vi "rad_Format Image Results.vi"(7 "Results listbox":refnum<vi>, 8 "error in (no error)":errorcluster, 10 "AppImage 2":T1, 11 "AppImage 1":T1) -> (0 "error out":errorcluster)   [LabVIEW 2016]
uses:
  App Images/TypeDefs/rad_Application Image Properties.ctl
  App Images/TypeDefs/rad_FPGA Properties.ctl
  App Images/TypeDefs/rad_FPGA Flash Properties.ctl
  <vilib>/Utility/miscctls.llb/LVRowAndColumnTypeDef.ctl
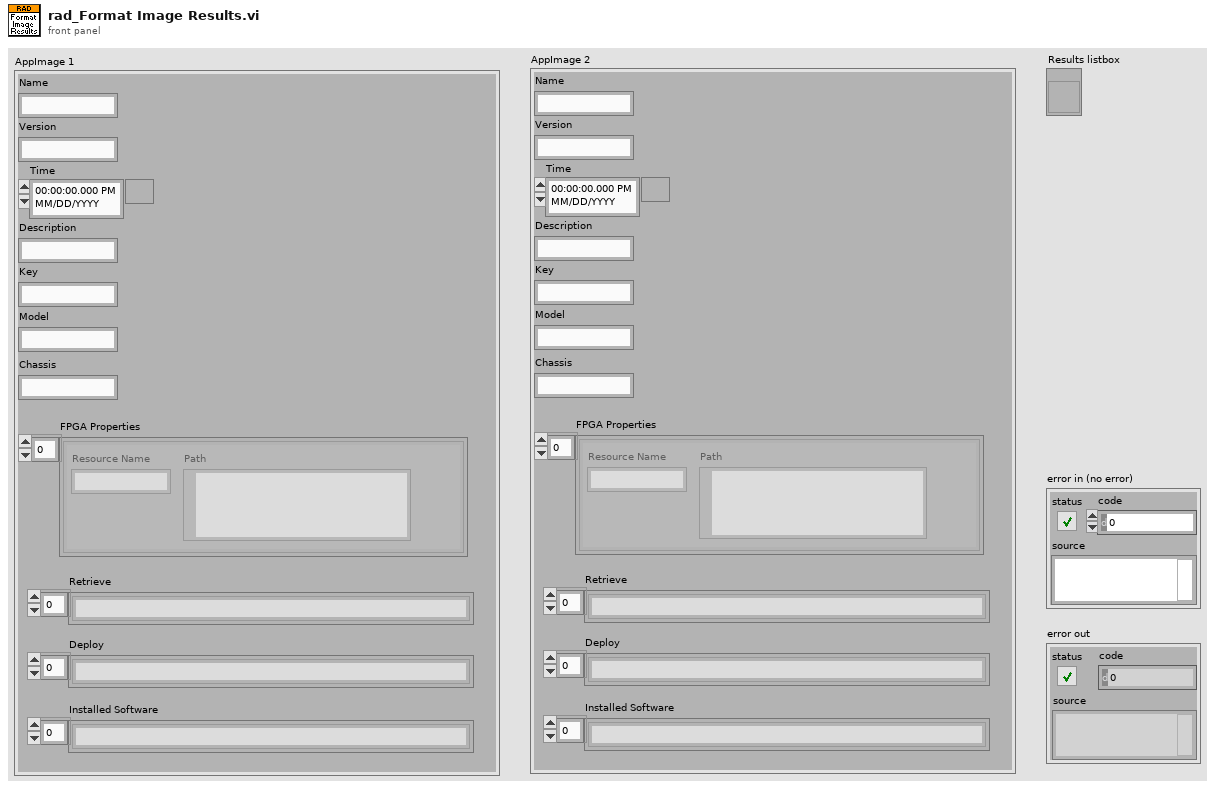
[diagram p1: front panel]
types:
  T1 = typedef "rad_Application Image Properties.ctl" = cluster{"Name":string, "Version":string, "Time":timestamp, "Description":string, "Key":string, "Chassis":string, "FPGA Properties":T2, "Model":string, "Retrieve":string[], "Deploy":string[], "Installed Software":string[]}
  T2 = typedef "rad_FPGA Properties.ctl" = T3[]
  T3 = typedef "rad_FPGA Flash Properties.ctl" = cluster{"Resource Name":string, "Path":path}
  T4 = typedef "LVRowAndColumnTypeDef.ctl" = cluster{"Row":i32, "Column":i32}
  T5 = cluster{"Name":string, "Version":string, "Matched":enum16{"Not matched", "Different version", "Same version"}}[]
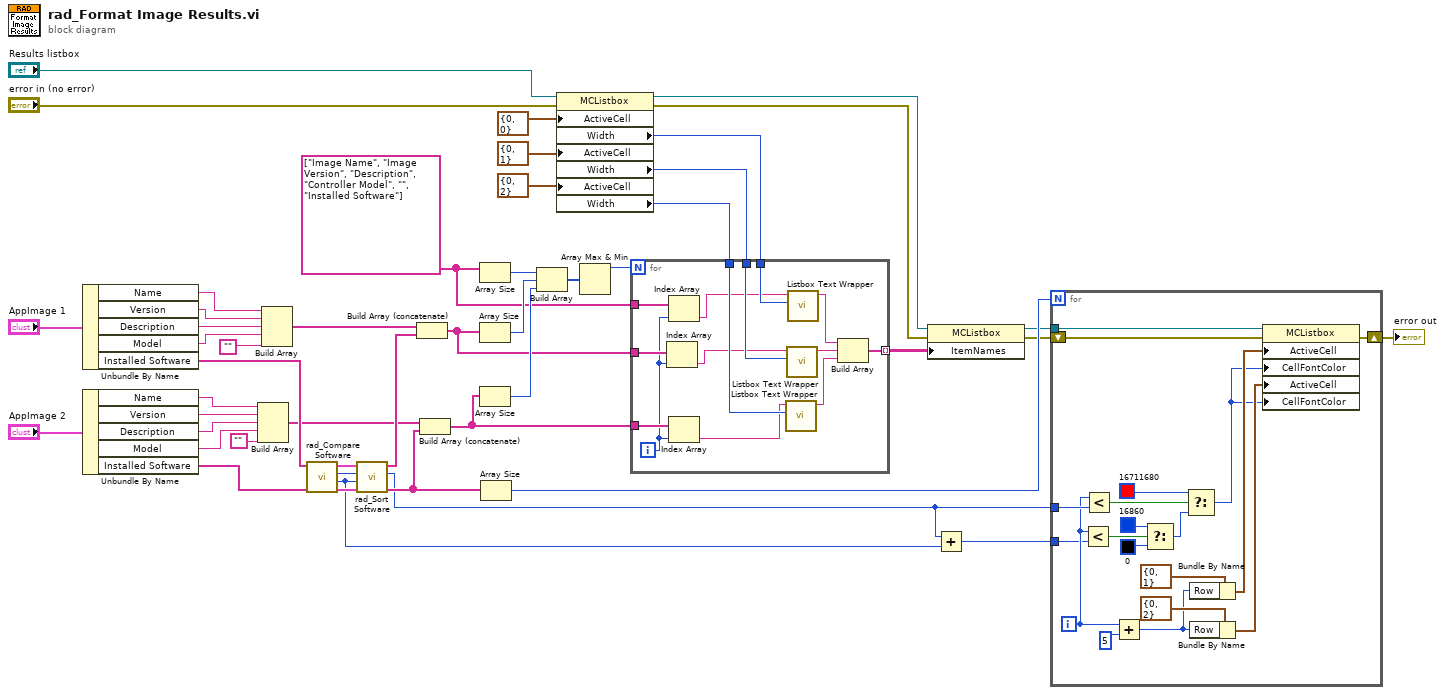
[diagram p0: block diagram]
diagram:
  w35 = string[] ["Image Name", "Image Version", "Description", "Controller Model", "", "Installed Software"]
  n1 = Unbundle By Name("AppImage 1") -> ("Name"=w25:string, "Version"=w26:string, "Description"=w27:string, "Model"=w28:string, "Installed Software"=w17:string[])
  n2 = Unbundle By Name("AppImage 2") -> ("Name"=w24:string, "Version"=w23:string, "Description"=w22:string, "Model"=w21:string, "Installed Software"=w16:string[])
  n3 = Build Array(w24, w23, w22, w21, "") -> (w11:string[])
  n4 = Build Array(w25, w26, w27, w28, "") -> (w18:string[])
  n5 = call "rad_Compare Software.vi"("Installed Software 2"=w16, "Installed Software 1"=w17) -> ("Analyzed Software 2"=w14:T5, "Different version"=w2:i32, "Same version"=w9:i32, "Analyzed Software 1"=w15:T5)  [unwired: 6 in]
  n6 = call "rad_Sort Software.vi"("Analyzed Software 2"=w14, "Different version"=w2, "Same version"=w9, "Analyzed Software 1"=w15) -> ("Sorted Software 2"=w8:string[], "Not matched"=w3:i32, "Sorted Software 1"=w12:string[])  [unwired: 5 in]
  n7 = Build Array (concatenate)(w18, w12) -> (w13:string[])
  n8 = Build Array (concatenate)(w11, w8) -> (w10:string[])
  n9 = Array Size(array=w35) -> (size(s)=w47:i32)
  n10 = Array Size(array=w13) -> (size(s)=w46:i32)
  n11 = Array Size(array=w10) -> (size(s)=w45:i32)
  n12 = Array Size(array=w8) -> (size(s)=w7:i32)
  n13 = Build Array(w47, w46, w45) -> (w44:i32[])
  n14 = property on="Property Node" class="MCListbox"(reference="Results listbox", error in="error in (no error)", "ActiveCell"=T4 {"Row"=0, "Column"=0} ("Active Cell:Active Cell"), "ActiveCell"=T4 {"Row"=0, "Column"=1} ("Active Cell:Active Cell"), "ActiveCell"=T4 {"Row"=0, "Column"=2} ("Active Cell:Active Cell")) -> (reference out=w33:refnum<vi>, error out=w32:errorcluster, "Width"=w39:u32, "Width"=w38:u32, "Width"=w37:u32)
  n15 = Array Max & Min(array=w44) -> (max value=w43:i32)  [unwired: 3 out]
  n16 = for {
    N: w43 -> [_]
    tunnel: w35 -> [w61]
    tunnel: w13 -> [w60]
    tunnel: w10 -> [w59]
    tunnel: [w57] -> w36 mode=indexing
    tunnel: w39 -> [w56]
    tunnel: w38 -> [w55]
    tunnel: w37 -> [w54]
    i -> [w58]
    n17 = Index Array(array=w60, index=w58) -> (element=w52:string)
    n18 = Index Array(array=w61, index=w58) -> (element=w53:string)
    n19 = Index Array(array=w59, index=w58) -> (element=w51:string)
    n20 = call "Listbox Text Wrapper.vi"("Size:Width"=w54, "Input Text"=w51) -> ("Wrapped Text"=w50:string)  [unwired: 9 in]
    n21 = call "Listbox Text Wrapper.vi"("Size:Width"=w55, "Input Text"=w52) -> ("Wrapped Text"=w49:string)  [unwired: 9 in]
    n22 = call "Listbox Text Wrapper.vi"("Size:Width"=w56, "Input Text"=w53) -> ("Wrapped Text"=w48:string)  [unwired: 9 in]
    n23 = Build Array(w48, w49, w50) -> (w57:string[])
  }
  n24 = property class="MCListbox"(reference=w33, error in=w32, "ItemNames"=w36) -> (reference out=w6:refnum<vi>, error out=w5:errorcluster)
  n25 = Add(x=w3, y=w2) -> (x+y=w1:i32)
  n26 = for {
    N: w7 -> [_]
    tunnel: w6 -> [w79]
    shift-right: [w78] -> w4
    shift-left: w5 -> [w80]
    tunnel: w3 -> [w73]
    tunnel: w1 -> [w69]
    i -> [w70]
    n27 = Less?(x=w70, y=w69) -> (x < y?=w68:bool)
    n28 = Less?(x=w70, y=w73) -> (x < y?=w72:bool)
    n29 = Add(x=w70, y=5) -> (x+y=w63:i32)
    n30 = Select(t=u32 16860, s=w68, f=u32 0) -> (s? t:f=w65:u32)
    n31 = Select(t=u32 16711680, s=w72, f=w65) -> (s? t:f=w64:u32)
    n32 = Bundle By Name(cluster=T4 {"Row"=0, "Column"=1} ("Active Cell:Active Cell"), "Row"=w63) -> (w75:T4)
    n33 = Bundle By Name(cluster=T4 {"Row"=0, "Column"=2} ("Active Cell:Active Cell"), "Row"=w63) -> (w74:T4)
    n34 = property class="MCListbox"(reference=w79, error in=w80, "ActiveCell"=w75, "CellFontColor"=w64, "ActiveCell"=w74, "CellFontColor"=w64) -> (error out=w78:errorcluster)  [unwired: 1 out]
  }
  "error out" <- w4
